vi "GUI_laptop v3.vi"() -> ()   [LabVIEW 2019]
uses:
  <vilib>/Math Plots/3D Math Plots/3D Scatter/3D Scatter XCtrl/3D Scatter.xctl
  <vilib>/Platform/TimedLoop/XDataNode/timing_clust.ctl
  <vilib>/Platform/TimedLoop/XDataNode/nitl_modes.ctl
  <vilib>/Platform/TimedLoop/XDataNode/wakeup.ctl
  <vilib>/Analysis/_algsub.llb/Real Vector Norm.vi
  <vilib>/Instr/_visa.llb/VISA Configure Serial Port (Instr).vi
  <vilib>/Math Plots/3D Math Plots/3D Scatter/3D Scatter Datatype/Public/Plot Helper (Vector).vi
  <vilib>/Utility/file.llb/Write Delimited Spreadsheet (DBL).vi
  <vilib>/platform/TimedLoop/XDataNode/XDataNode.xnode
  <vilib>/Platform/TimedLoop/XDataNode/XDNodeRunTimeDep.lvlib
  <vilib>/Math Plots/3D Math Plots/3D Scatter/3D Scatter Datatype/3D Scatter Datatype.lvclass
  <vilib>/Analysis/NI_AALPro.lvlib
panel:
  out "Finished Late? [i-1]":bool
  in  "Epsilon":dbl=0.2
  out "3D Scatter":refnum<class "3D Plot Datatype.lvclass">[](xcontrol)
  out "Random Point":dbl[](array[numeric])
  out "Virtual Cursor":dbl[](array[numeric])
  out "Iteration Duration":i64
  in  "Num of Points":i32=10
  in  "z bound":dbl=2.0
  in  "y bound":dbl=5.0
  in  "x bound":dbl=5.0
  in  "Stop":bool
  in  "Round Decimals":dbl=2.0 format="%#_15g"
  in  "Save  Data":bool
  in  "Save Path":path
  in  "x speed":dbl=0.5
  in  "z speed":dbl=0.5
  in  "y speed":dbl=0.5
  out "error out":errorcluster
  in  "baud rate":u32=115200
  in  "VISA resource name":refnum<visa-resource-name>
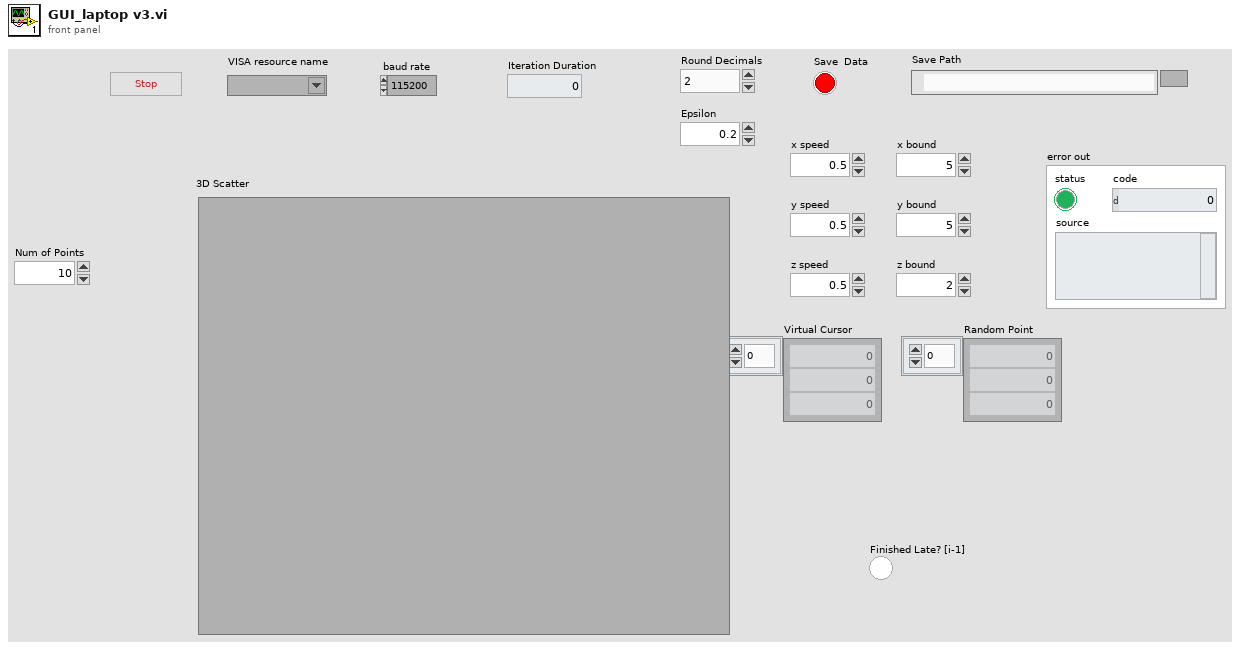
[diagram p1: front panel]
types:
  T1 = typedef "XDNodeRunTimeDep.lvlib/timing_clust.ctl" = cluster{"Expected End [f-1]":u64, "Actual End [f-1]":u64, "Finished Late? [f-1]":bool, "Expected End [i-1]":u64, "Actual End [i-1]":u64, "Finished Late? [i-1]":bool, "Expected Start [i]":u64, "Actual Start [i]":u64, "Expected Start [f]":u64, "Actual Start [f]":u64, "Source Name":string, "Structure Name":string, "Period":i64, "Deadline":i64, "Offset":i64, "Start":i64, "Priority":i32, "Timeout":i32, "Mode":T2, "Wakeup Reason":T3, "Error":errorcluster, "Source Type":string, "Secondary Source Type":string, "Global End Time":u64, "Global Start Time":u64, "Frame Duration":u64, "Iteration Duration":u64, "Assigned CPU":i32, "I/O Scan Engine Mode":u32}
  T2 = typedef "XDNodeRunTimeDep.lvlib/nitl_modes.ctl" = enum32{"No Change", "Process missed periods, maintain original phase", "Discard missed periods, maintain original phase", "Process missed periods, ignore original phase", "Discard missed periods, ignore original phase"}
  T3 = typedef "XDNodeRunTimeDep.lvlib/wakeup.ctl" = enum32{"Normal", "Aborted", "Asynchronous wakeup", "Timing source error", "Timed loop error", "Timeout"}
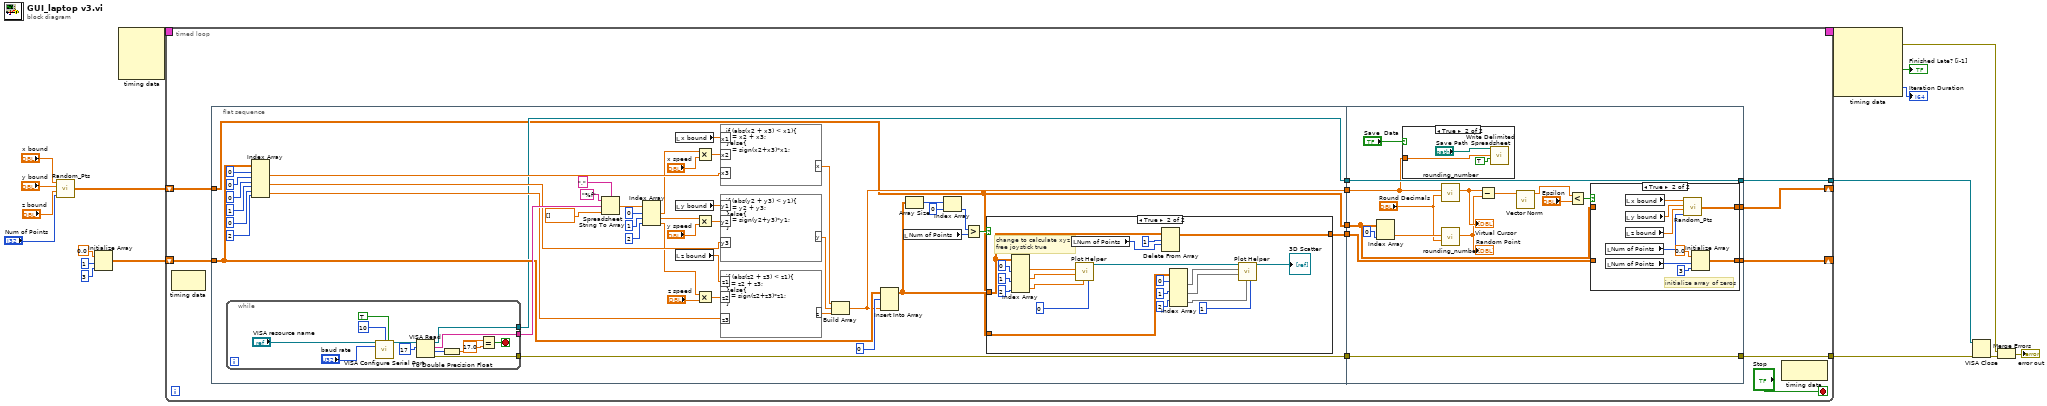
[diagram p0: block diagram]
diagram:
  n1 = call "Random_Pts.vi"("Num of Points"="Num of Points", "z bound"="z bound", "y bound"="y bound", "x bound"="x bound") -> ("appended array"=w4:dbl[][])
  n2 = Initialize Array(0.0 ("element"), 1 ("dimension size"), 3 ("dimension size")) -> (w11:dbl[][])
  n3 = node-c288() -> (w18:T1)  [unwired: 4 in]
  n4 = timed-loop {
    tunnel: [w29] -> w13
    tunnel: [w28] -> w12
    shift-right: [w27] -> _
    shift-left: w11 -> [w26]
    timing: w18 -> [_]
    timing-out: [_] -> w17
    shift-right: [w19] -> _
    shift-left: w4 -> [w21]
    stop <- "Stop" stop-if-true
    n5 = node-c288() -> ()  [unwired: 1 in, 1 out]
    n6 = flat-sequence {
      tunnel: w26 -> [w50]
      tunnel: [w37] -> w25
      tunnel: [w74] -> w24
      tunnel: [w39] -> w23
      tunnel: [w43] -> w22
      tunnel: w21 -> [w33]
      tunnel: [w33] -> w20
      tunnel: w25 -> [w129]
      tunnel: w24 -> [w128]
      tunnel: w23 -> [w121]
      tunnel: w22 -> [w123]
      tunnel: w20 -> [w125]
      tunnel: [w129] -> w29
      tunnel: [w128] -> w28
      tunnel: [w120] -> w27
      tunnel: [w124] -> w19
      frame #0 {
        n7 = while {
          tunnel: [w111] -> w77
          tunnel: [w106] -> w74
          tunnel: [w100] -> w37
          stop <- w110 stop-if-true
          n8 = call-poly "VISA Configure Serial Port"("VISA resource name"="VISA resource name", "termination char\n(0xA = '\\n' = LF)"=u8 10 ("termination char\n(0xA = '\\n' = LF)"), "Enable Termination\nChar (T)"=TRUE ("Enable Termination\nChar (T)"), "baud rate (9600)"="baud rate") -> ("VISA resource name out"=w101:refnum<visa-resource-name>)  [unwired: 10 in, 1 out]
          n9 = VISA Read(VISA resource name=w101, byte count=u32 17) -> (VISA resource name out=w100:refnum<visa-resource-name>, read buffer=w111:string, return count=w108:u32, error out=w106:errorcluster)  [unwired: 1 in]
          n10 = To Double Precision Float(number=w108) -> (double precision float=w107:dbl)
          n11 = Equal?(x=w107, y=17.0 ("char count")) -> (x = y?=w110:bool)
        }
        n12 = Index Array(array=w50, index (row) #1=0 ("disabled index (row)"), index (col) #1=0 ("disabled index (col)"), index (row) #2=0 ("disabled index (row)"), index (col) #2=1 ("disabled index (col)"), index (row) #3=0 ("disabled index (row)"), index (col) #3=2 ("disabled index (col)")) -> (element #1=w64:dbl, element #2=w58:dbl, element #3=w61:dbl)
        n13 = Spreadsheet String To Array(delimiter (Tab)=",", format string="%f", spreadsheet string=w77, array type (2D Dbl)=dbl[] []) -> (array=w38:dbl[])
        n14 = Index Array(array=w38, index #1=0 ("index"), index #2=1 ("index"), index #3=2 ("index")) -> (element #1=w36:dbl, element #2=w35:dbl, element #3=w34:dbl)
        n15 = local read "x bound"() -> (w46:dbl)
        n16 = local read "y bound"() -> (w45:dbl)
        n17 = local read "z bound"() -> (w44:dbl)
        n18 = Multiply(x=w36, y="x speed") -> (x*y=w65:dbl)
        n19 = Multiply(x=w35, y="y speed") -> (x*y=w60:dbl)
        n20 = Multiply(x=w34, y="z speed") -> (x*y=w62:dbl)
        n21 = formula code="if (abs(x2 + x3) < x1){\nx = x2 + x3;\n}else{\nx = sign(x2+x3)*x1;\n}"("x1"=w46, "x2"=w65, "x3"=w64) -> ("x"=w54:dbl)
        n22 = formula code="if (abs(y2 + y3) < y1){\ny = y2 + y3;\n}else{\ny = sign(y2+y3)*y1;\n}"("y1"=w45, "y2"=w60, "y3"=w58) -> ("y"=w52:dbl)
        n23 = formula code="if (abs(z2 + z3) < z1){\nz = z2 + z3;\n}else{\nz = sign(z2+z3)*z1;\n}"("z1"=w44, "z2"=w62, "z3"=w61) -> ("z"=w53:dbl)
        n24 = Build Array(w54, w52, w53) -> (w43:dbl[])
        n25 = Insert Into Array(array=w50, index (row)=0, new element=w43) -> (w41:dbl[][])  [unwired: 1 in]
        n26 = local read "Num of Points"() -> (w42:i32)
        n27 = Array Size(array=w41) -> (size(s)=w51:i32[])
        n28 = Index Array(array=w51, index=0) -> (element=w55:i32)
        n29 = Greater?(x=w55, y=w42) -> (0:w40:bool)
        n30 = case shown="True" w40 {
          tunnel: w41 -> [w78 w95]
          tunnel: [w78 w94] -> w39
          tunnel: w33 -> [_ w93]
          frame False {
          }
          frame True {
            # "change to calculate xyz if \nfree joystick true"
            n31 = Index Array(array=w95, index (col) #1=0 ("disabled index (col)"), index (col) #2=1 ("index (col)"), index (col) #3=2 ("index (col)")) -> (element #1=w84:dbl[], element #2=w83:dbl[], element #3=w82:dbl[])  [unwired: 3 in]
            n32 = local read "Num of Points"() -> (w92:i32)
            n33 = call-poly <vilib>:"Plot Helper.vi"("Plot ID"=0, "z vector"=w82, "y vector"=w83, "x vector"=w84) -> ("3D Plot lvclass Array out"=w86:refnum<class "3D Plot Datatype.lvclass">[])  [unwired: 2 in, 5 out]
            n34 = Delete From Array(array=w95, length=1, index (row)=w92) -> (array with subset deleted=w94:dbl[][])  [unwired: 1 in, 1 out]
            n35 = Index Array(array=w93, index (row) #1=0 ("index (row)"), index (row) #2=1 ("index (row)"), index (row) #3=2 ("index (row)")) -> (element #1=w90:dbl[], element #2=w89:dbl[], element #3=w88:dbl[])  [unwired: 3 in]
            n36 = call-poly <vilib>:"Plot Helper.vi"("Plot ID"=1, "z vector"=w88, "y vector"=w89, "x vector"=w90, "3D Plot lvclass Array in"=w86) -> ("3D Plot lvclass Array out"=→"3D Scatter":refnum<class "3D Plot Datatype.lvclass">[])  [unwired: 1 in, 5 out]
          }
        }
      }
      frame #1 {
        n37 = Index Array(array=w125, index (col)=0 ("index (row)")) -> (element=w127:dbl[])  [unwired: 1 in]
        n38 = case shown="True" "Save  Data" {
          tunnel: w123 -> [_ w130]
          frame False {
          }
          frame True {
            n39 = call-poly <vilib>:"Write Delimited Spreadsheet.vi"("file path (dialog if empty)"="Save Path", "1D data"=w130, "append to file? (new file:F)"=TRUE) -> ()  [unwired: 11 in, 2 out]
          }
        }
        n40 = call "rounding_number.vi"("power of ten"="Round Decimals", "Array"=w123) -> ("rounded"=w119:dbl[])  [unwired: 9 in]
        "Virtual Cursor" <- w119
        n41 = call "rounding_number.vi"("power of ten"="Round Decimals", "Array"=w127) -> ("rounded"=w118:dbl[])  [unwired: 9 in]
        "Random Point" <- w118
        n42 = Subtract(x=w119, y=w118) -> (x-y=w117:dbl[])
        n43 = call-poly <vilib>:"Vector Norm.vi"("Input Vector"=w117) -> ("norm"=w116:dbl)  [unwired: 9 in, 1 out]
        n44 = Less?(x=w116, y="Epsilon") -> (x < y?=w114:bool)
        n45 = case shown="True" w114 {
          tunnel: w125 -> [w134 _]
          tunnel: [w134 w139] -> w124
          tunnel: w121 -> [w133 _]
          tunnel: [w133 w135] -> w120
          frame False {
          }
          frame True {
            # "initialize array of zeros"
            n46 = local read "Num of Points"() -> (w140:i32)
            n47 = local read "Num of Points"() -> (w137:i32)
            n48 = local read "x bound"() -> (w143:dbl)
            n49 = local read "y bound"() -> (w142:dbl)
            n50 = local read "z bound"() -> (w141:dbl)
            n51 = call "Random_Pts.vi"("Num of Points"=w140, "z bound"=w141, "y bound"=w142, "x bound"=w143) -> ("appended array"=w139:dbl[][])
            n52 = Initialize Array(0.0 ("element"), w137, 3 ("dimension size")) -> (w135:dbl[][])
          }
        }
      }
    }
    n53 = node-c288() -> ()  [unwired: 1 in, 1 out]
  }
  n54 = node-c288(w17) -> (w10:errorcluster, →"Finished Late? [i-1]":bool, →"Iteration Duration":i64)  [unwired: 3 out]
  n55 = VISA Close(VISA resource name=w13, error in (no error)=w12) -> (error out=w9:errorcluster)
  n56 = Merge Errors(w10, w9) -> (→"error out":errorcluster)
